vi "Edge Detector.vi"(1 "Input":bool) -> (0 "Rising / falling edge?":bool)   [LabVIEW 2014]
doc: "Return true if the input changed from true to false.\n\nInlined."
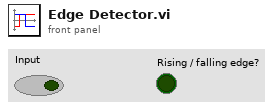
[diagram p1: front panel]
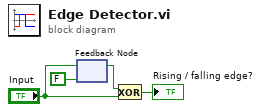
[diagram p0: block diagram]
diagram:
  n1 = feedback #1(FALSE ("Input")) -> (w3:bool)
  n2 = feedback-in #1("Input") -> ()
  n3 = Exclusive Or(1:"Input", 2:w3) -> (0:→"Rising / falling edge?":bool)
